vi "Read Actor Info.vi"(8 "Error In":errorcluster, 11 "CS++Factory in":refnum<class "CS++Factory.lvclass">) -> (0 "Error Out":errorcluster, 2 "Actors":cluster{"Name":string, "LVClassPath":string}[](array[cluster]), 3 "CS++Factory out":refnum<class "CS++Factory.lvclass">)   [LabVIEW 2016, in "CS++BaseClasses.lvlib" / "CS++Factory.lvclass"]
doc: "Read object attribute data from storage medium.\n\nThe default implementation reads from ini-file."
uses:
  CS++Factory.lvclass
  CS++Factory.lvclass/CS++Factory.ctl
  <vilib>/ActorFramework/Actor/Actor.lvclass
  <vilib>/Utility/config.llb/Read Key (String).vi
  <vilib>/Utility/config.llb/NI_LVConfig.lvlib
  Libraries/Utilities/CS++Utilities.lvlib
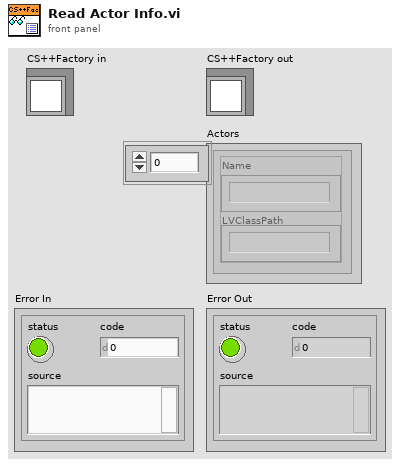
[diagram p1: front panel]
types:
  T1 = typedef "NI_LVConfig.lvlib/Config Data RefNum.ctl" = refnum<k1>
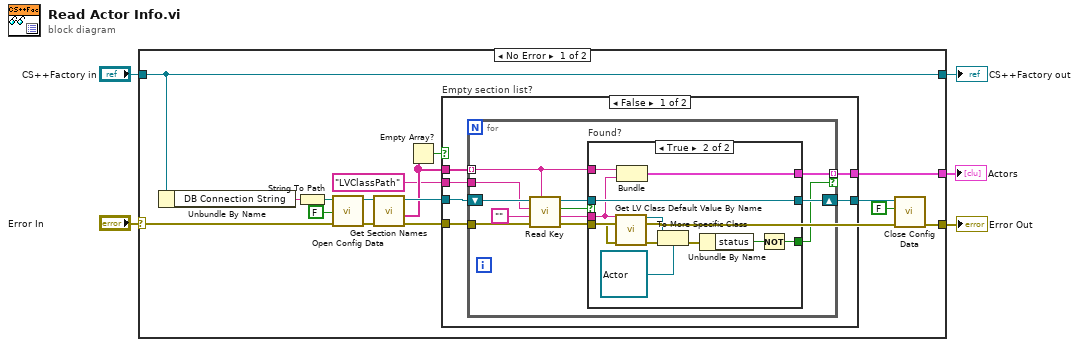
[diagram p0: block diagram]
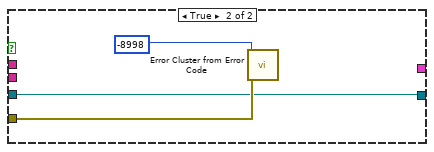
[diagram p3: hidden frame]
diagram:
  n1 = case shown="No Error" "Error In" {
    selector: "Error In" -> [w15 w56]
    tunnel: [w14 w56] -> w4
    tunnel: [w21 w55] -> w2
    tunnel: "CS++Factory in" -> [w21 w55]
    tunnel: [w7 _] -> w1
    frame No Error {
      n2 = Unbundle By Name(w21) -> ("DB Connection String"=w10:string)
      n3 = String To Path(string=w10) -> (path=w11:path)
      n4 = call <vilib>:"Open Config Data.vi"("error in (no error)"=w15, "create file if necessary (T)"=FALSE, "configuration file path"=w11) -> ("error out"=w17:errorcluster, "refnum"=w18:T1)  [unwired: 6 in, 1 out]
      n5 = call <vilib>:"Get Section Names.vi"("error in (no error)"=w17, "refnum"=w18) -> ("error out"=w6:errorcluster, "section names"=w13:string[], "refnum out"=w16:T1)  [unwired: 7 in]
      n6 = Empty Array?(array=w13) -> (empty?=w9:bool)
      n7 = case "Empty section list?" shown="False" w9 {
        tunnel: [w27 w52] -> w20
        tunnel: w6 -> [w24 w54]
        tunnel: w16 -> [w26 w52]
        tunnel: w13 -> [w25 _]
        tunnel: "LVClassPath" -> [w23 _]
        tunnel: [w22 _] -> w7
        frame False {
          n8 = for {
            tunnel: w25 -> [w29] mode=indexing
            shift-right: [w33] -> w27
            shift-left: w26 -> [w39]
            tunnel: w23 -> [w37]
            tunnel: [w28] -> w22 mode=indexing if=w30
            tunnel: w24 -> [w38]
            n9 = call-poly <vilib>:"Read Key.vi"("section"=w29, "error in (no error)"=w38, "default value"="", "key"=w37, "refnum"=w39) -> ("error out"=w34:errorcluster, "value"=w35:string, "found?"=w31:bool, "refnum out"=w32:T1)  [unwired: 3 in]
            n10 = case "Found?" shown="True" w31 {
              tunnel: w35 -> [_ w43]
              tunnel: [w40 w50] -> w33
              tunnel: w32 -> [w40 w50]
              tunnel: w34 -> [_ w51]
              tunnel: [_ w41] -> w30
              tunnel: w29 -> [_ w44]
              tunnel: [_ w42] -> w28
              frame False {
              }
              frame True {
                n11 = call <vilib>:"Get LV Class Default Value By Name.vi"("error in (no error)"=w51, "class name"=w43) -> ("error out"=w48:errorcluster, "object"=w49:refnum<class>)  [unwired: 8 in]
                n12 = Bundle("String"=w44, "value"=w43) -> (w42:cluster{"String":string, "value":string})  [unwired: 1 in]
                n13 = To More Specific Class(target class=refnum<class "Actor.lvclass"> refnum ("Actor Framework:Actor"), reference=w49, error in=w48) -> (error out=w46:errorcluster)  [unwired: 1 out]
                n14 = Unbundle By Name(w46) -> ("status"=w45:bool)
                n15 = Not(x=w45) -> (.not. x?=w41:bool)
              }
            }
          }
        }
        frame True {
          n16 = call "Error Cluster from Error Code.vi"("Error In"=w54, "Error Code (0)"=-8998 ("Object configuration data not found")) -> ()  [unwired: 9 in, 1 out]
        }
      }
      n17 = call <vilib>:"Close Config Data.vi"("error in (no error)"=w6, "write file if changed (T)"=FALSE, "refnum"=w20) -> ("error out"=w14:errorcluster)  [unwired: 7 in, 1 out]
    }
    frame Error {
    }
  }
  "Error Out" <- w4
  "CS++Factory out" <- w2
  "Actors" <- w1
